vi "Post-Build Action_EditExeIniFile_Allowmultipleinstances.vi"(5 "Files Generated by Build":path[](array[path]), 6 "Top Level/Always Included VIs":path[](array[path]), 7 "Destination Path":path, 8 "error in (no error)":errorcluster, 9 "Target Name":string, 10 "Build Specification Name":string, 11 "Project Path":path) -> (0 "error out":errorcluster)   [LabVIEW 2021]
uses:
  <vilib>/Utility/config.llb/NI_LVConfig.lvlib
  <vilib>/Utility/config.llb/Write Key (String).vi
panel:
  out "error out 2":errorcluster
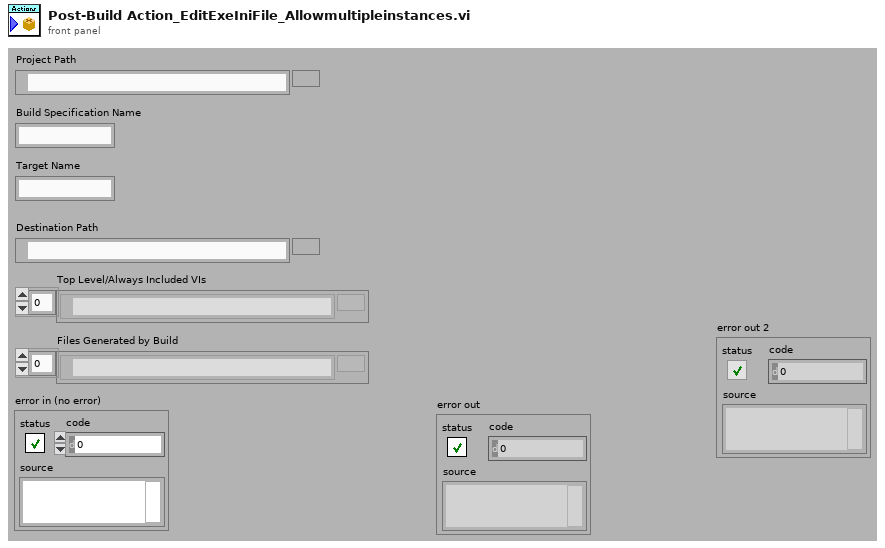
[diagram p1: front panel]
types:
  T1 = typedef "NI_LVConfig.lvlib/Config Data RefNum.ctl" = refnum<k1>
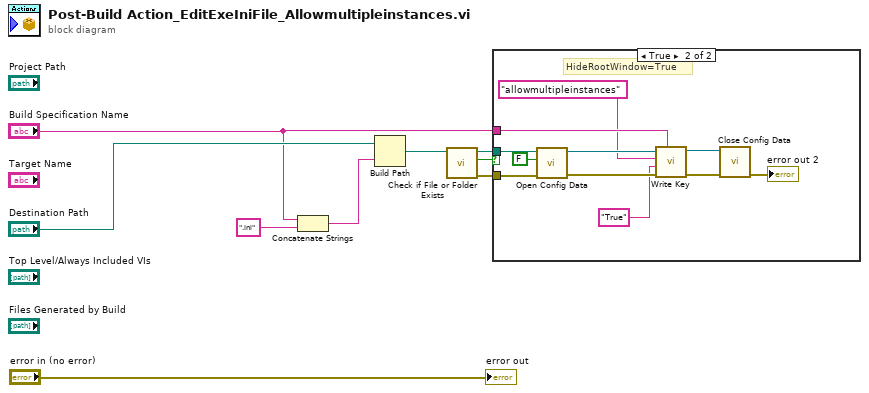
[diagram p0: block diagram]
diagram:
  n1 = Concatenate Strings("Build Specification Name", ".ini" ("string")) -> (w4:string)
  n2 = Build Path(base path="Destination Path", name or relative path=w4) -> (appended path=w5:path)
  n3 = call <vilib>:"Check if File or Folder Exists.vi"("path"=w5) -> ("error out"=w7:errorcluster, "file or folder exists?"=w8:bool, "dup path"=w6:path)  [unwired: 8 in]
  n4 = case shown="True" w8 {
    tunnel: w6 -> [_ w20]
    tunnel: w7 -> [_ w19]
    tunnel: "Build Specification Name" -> [_ w15]
    frame False {
    }
    frame True {
      # "HideRootWindow=True"
      n5 = call <vilib>:"Open Config Data.vi"("error in (no error)"=w19, "create file if necessary (T)"=FALSE, "configuration file path"=w20) -> ("error out"=w16:errorcluster, "refnum"=w17:T1)  [unwired: 6 in, 1 out]
      n6 = call-poly <vilib>:"Write Key.vi"("section"=w15, "error in (no error)"=w16, "value"="True" ("key"), "key"="allowmultipleinstances", "refnum"=w17) -> ("error out"=w11:errorcluster, "refnum out"=w12:T1)  [unwired: 4 in, 1 out]
      n7 = call <vilib>:"Close Config Data.vi"("error in (no error)"=w11, "refnum"=w12) -> ("error out"=→"error out 2":errorcluster)  [unwired: 8 in, 1 out]
    }
  }
  "error out" <- "error in (no error)"
